vi "GetLinkerDependencyFromFiles.vi"(9 "Overwrite LabVIEW Folder(If empty use this version of LabVIEW)":path, 10 "MaxDepth(<=0 No limit)":i32=-1, 11 "All Files in Dir":path[](array[path])) -> (3 "FileDependency":map{path, T1}(c390))   [LabVIEW 2020, in "DependencyViewer.lvlib"]
uses:
  DependencyViewer.lvlib
  FileDependencyType.ctl
  <vilib>/Utility/lvfile.llb/FT_FileTypes.ctl
  fa84a50a-7a91-41f1-93a7-6c8b41b91fd3.vi
  <vilib>/Utility/lvfile.llb/NI_FileType.lvlib
panel:
  out "Dependecy":T1
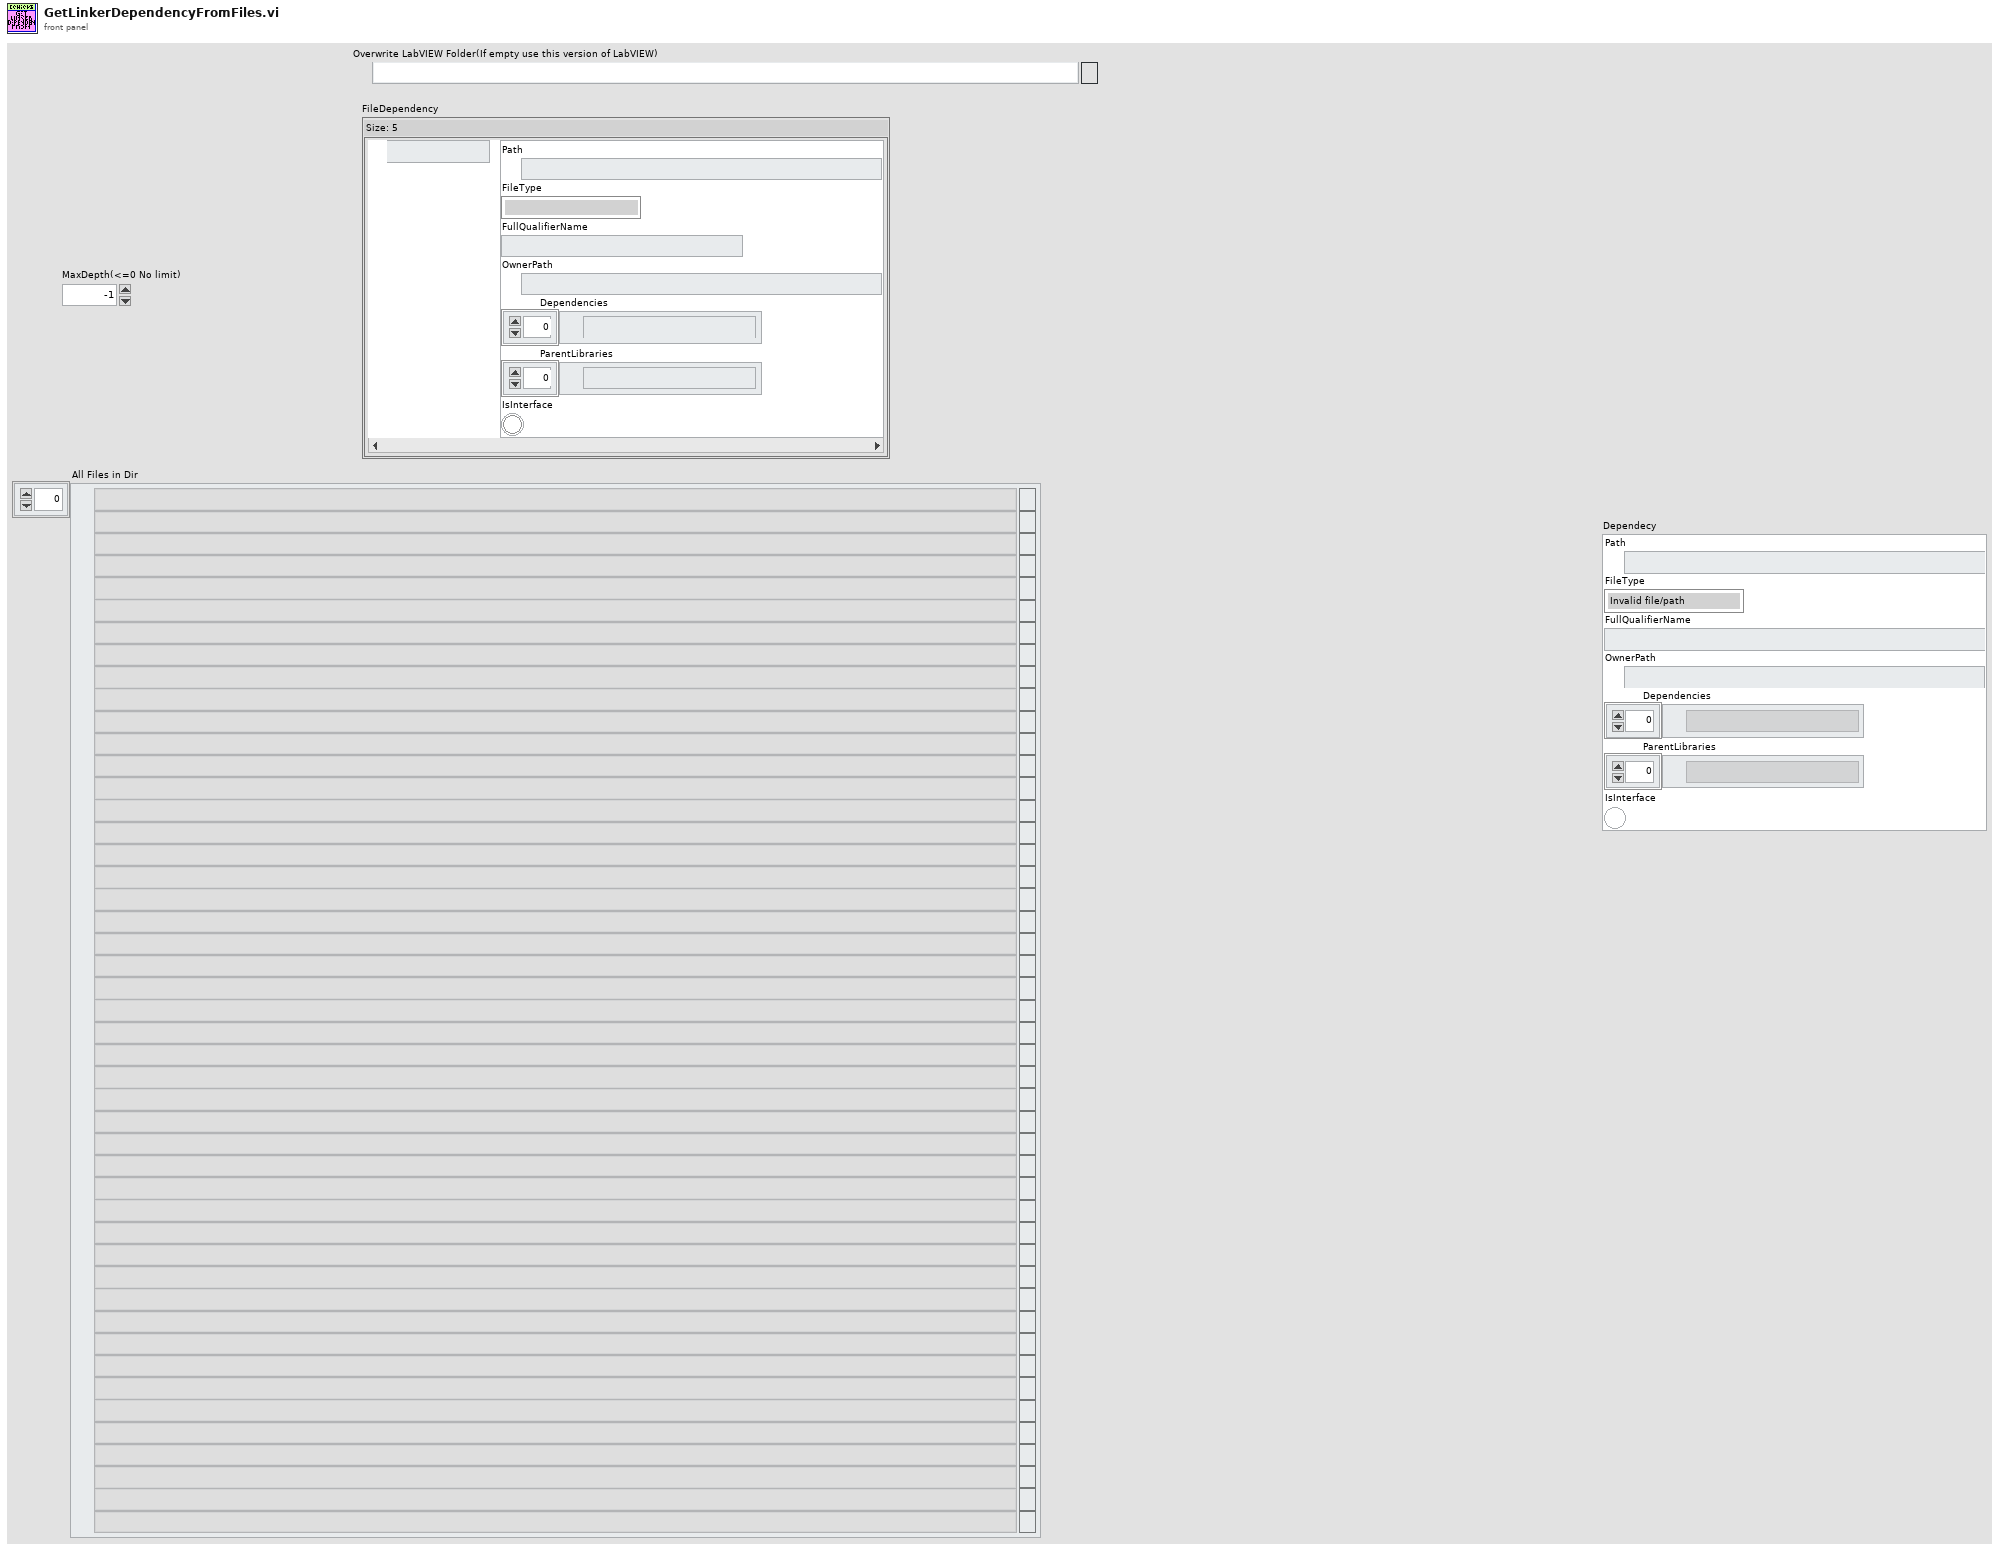
[diagram p1: front panel]
types:
  T1 = typedef "DependencyViewer.lvlib/FileDependencyType.ctl" = cluster{"Path":path, "FileType":T2, "FullQualifierName":string, "OwnerPath":path, "Dependencies":path[], "ParentLibraries":path[], "IsInterface":bool}
  T2 = typedef "NI_FileType.lvlib/FT_FileTypes.ctl" = enum32{"Invalid file/path", "Unknown type", "Instrument", "Control", "Polymorphic VI", "Project", "Library", "LVClass", "XControl", "XNode", "CIN", "Run-time menu", "Palette menu", "LLB", "Shortcut", "Directory", "Class Private Data Control", "Statechart", "MathScript .m file", "Ladder Diagram", "LVLibp"}
  T3 = typedef "NI_FileType.lvlib/LVFileType.ctl" = enum32{"Invalid file", "Unknown type", "Instrument", "Control", "Polymorphic VI", "Project", "Library", "LVClass", "XControl", "XNode", "Shared library", ".NET assembly", "ActiveX interface", "CIN", "Run-time menu", "Palette menu", "Help file", "LLB", "XNode Edit Dependency", "Class Private Data Control", "Statechart", "MathScript .m file", "Ladder Diagram", "LVLibp", "XNode Build Dependency"}
  T4 = cluster{"path":path, "delimited name":string, "type":T3, "iState":u32, "iStyle":u16, "wStyle":u16, "buttons":u16, "viflags":u32, "viflags2":u32, "links":u32[]}[]
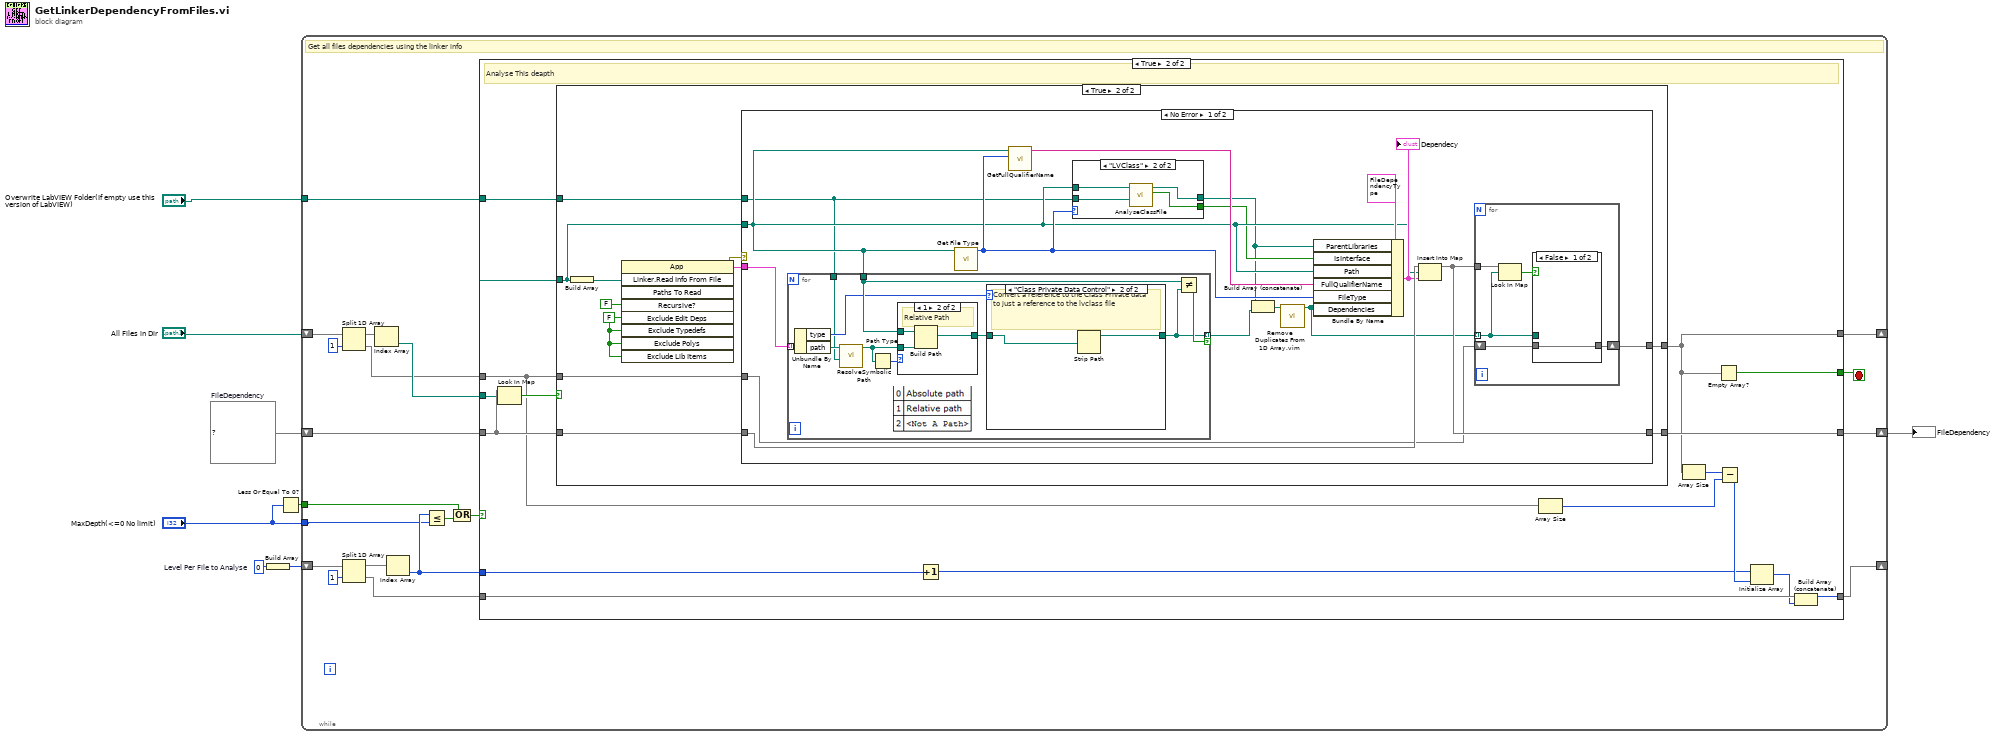
[diagram p0: block diagram]
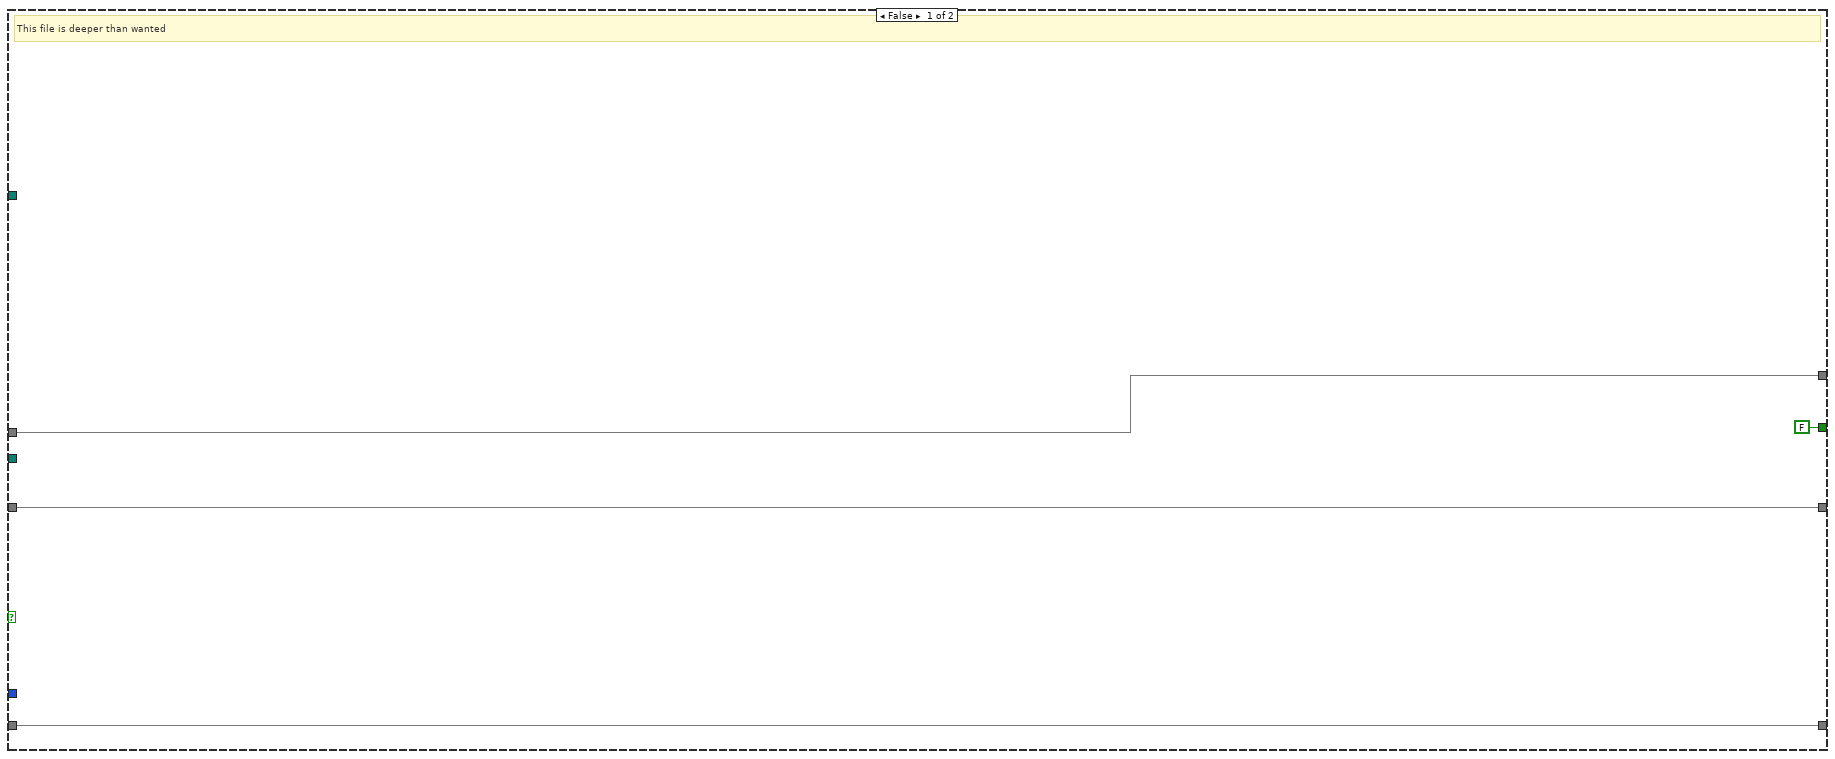
[diagram p2: hidden frame]
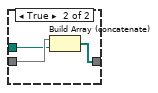
[diagram p5: hidden frame]
diagram:
  w4 = 0  # Level Per File to Analyse
  w7 = map{path, T1} {}  # FileDependency
  n1 = Build Array(w4) -> (w3:i32[])
  n2 = Less Or Equal To 0?(x="MaxDepth(<=0 No limit)") -> (x <= 0?=w1:bool)
  n3 = while {
    shift-right: [w25] -> w8
    shift-left: w7 -> [w24]
    shift-right: [w16] -> _
    shift-left: "All Files in Dir" -> [w28]
    tunnel: "Overwrite LabVIEW Folder(If empty use this version of LabVIEW)" -> [w22]
    tunnel: "MaxDepth(<=0 No limit)" -> [w12]
    shift-right: [w14] -> _
    shift-left: w3 -> [w20]
    tunnel: w1 -> [w9]
    stop <- w19 stop-if-true
    # "Get all files dependencies using the linker info"
    n4 = Split 1D Array(array=w28, index=1) -> (first subarray=w26:path[], second subarray=w17:path[])
    n5 = Split 1D Array(array=w20, index=1) -> (first subarray=w18:i32[], second subarray=w15:i32[])
    n6 = Index Array(array=w26) -> (element=w23:path)  [unwired: 1 in]
    n7 = Index Array(array=w18) -> (element=w13:i32)  [unwired: 1 in]
    n8 = Less Or Equal?(x=w13, y=w12) -> (x <= y?=w11:bool)
    n9 = Compound Arithmetic op=OR(w9, w11) -> (w10:bool)
    n10 = case shown="True" w10 {
      tunnel: [w30 w48] -> w25
      tunnel: w24 -> [w30 w47]
      tunnel: w23 -> [_ w45]
      tunnel: w22 -> [_ w44]
      tunnel: [FALSE ("empty?") w43] -> w19
      tunnel: w17 -> [w32 w42]
      tunnel: [w32 w41] -> w16
      tunnel: w15 -> [w31 w36]
      tunnel: [w31 w34] -> w14
      tunnel: w13 -> [_ w33]
      frame False {
        # "This file is deeper than wanted"
      }
      frame True {
        # "Analyse This deapth"
        n11 = Look In Map(map=w47, key=w45) -> (key not found?=w46:bool)  [unwired: 1 in, 1 out]
        n12 = case shown="True" w46 {
          tunnel: w42 -> [w49 w61]
          tunnel: [w50 w60] -> w48
          tunnel: [w49 w59] -> w41
          tunnel: w47 -> [w50 w54]
          tunnel: w45 -> [_ w53]
          tunnel: w44 -> [_ w51]
          frame False {
          }
          frame True {
            w52 = FALSE ("Exclude Edit Time Dependencies")
            n13 = Build Array(w53) -> (w58:path[])
            n14 = invoke class="App" method="Linker.Read Info From File"("Paths To Read"=w58, "Recursive?"=FALSE, "Exclude Edit Deps"=w52, "Exclude Typedefs"=w52, "Exclude Polys"=w52, "Exclude Lib Items"=w52) -> (error out=w55:errorcluster, "Linker.Read Info From File"=w56:T4)  [unwired: 3 in, 7 out]
            n15 = case shown="No Error" w55 {
              tunnel: w56 -> [w76 _]
              tunnel: w54 -> [w77 w108]
              tunnel: w61 -> [w73 w109]
              tunnel: [w72 w109] -> w59
              tunnel: w53 -> [w67 _]
              tunnel: [w74 w108] -> w60
              tunnel: w51 -> [w62 _]
              frame No Error {
                n16 = for {
                  tunnel: w76 -> [w100] mode=indexing
                  tunnel: [w92] -> w68 mode=indexing if=w97
                  tunnel: w67 -> [w96]
                  tunnel: w62 -> [w91]
                  n17 = Unbundle By Name(w100) -> ("type"=w94:T3, "path"=w98:path)
                  n18 = call "ResolveSymbolicPath.vi"("Overwrite LabVIEW Folder(If empty use this version of LabVIEW)"=w91, "path"=w98) -> ("File Path"=w95:path)  [unwired: 9 in]
                  n19 = Path Type(1:w95) -> (0:w99:i16)
                  n20 = case shown="1" w99 {
                    tunnel: w95 -> [w104 w107]
                    tunnel: [w104 w105] -> w93
                    tunnel: w96 -> [_ w106]
                    frame 0, Default {
                      # "Absolute Path"
                    }
                    frame 1 {
                      # "Relative Path"
                      n21 = Build Path(base path=w106, name or relative path=w107) -> (appended path=w105:path)
                    }
                  }
                  n22 = case shown="\"Class Private Data Control\"" w94 {
                    tunnel: w93 -> [w101 w103]
                    tunnel: [w101 w102] -> w92
                    frame Default {
                    }
                    frame "Class Private Data Control" {
                      # "Convert a reference to the Class Private data to just a reference to the lvclass file"
                      n23 = Strip Path(path=w103) -> (stripped path=w102:path)  [unwired: 1 out]
                    }
                  }
                  n24 = Not Equal?(x=w96, y=w92) -> (x != y?=w97:bool)
                }
                n25 = call <vilib>:"Get File Type.vi"("path"=w67) -> ("file type"=w70:T2)  [unwired: 8 in, 2 out]
                n26 = call "GetFullQualifierName.vi"("file type"=w70, "File Path"=w67) -> ("FullQualifierName"=w71:string)  [unwired: 9 in]
                n27 = case shown="\"LVClass\"" w70 {
                  tunnel: w67 -> [_ w81]
                  tunnel: [_ w80] -> w65
                  tunnel: [_ w79] -> w66
                  tunnel: w62 -> [_ w78]
                  frame "Invalid file/path", Default {
                  }
                  frame "LVClass" {
                    n28 = call "AnalyseClassFile.vi"("Overwrite LabVIEW Folder(If empty use this version of LabVIEW)"=w78, "File Path"=w81) -> ("IsInterface"=w79:bool, "ParentLibraries"=w80:path[])  [unwired: 8 in]
                  }
                }
                n29 = Build Array (concatenate)(w65, w68) -> (w64:path[])
                n30 = call "Remove Duplicates From 1D Array.vim"("array"=w64) -> ("array with duplicates removed"=w63:path[])  [unwired: 10 in]
                n31 = Bundle By Name(cluster=T1 {"Path"=path "", "FileType"=enum."Instrument", "FullQualifierName"="Decorator1_Main.vi", "OwnerPath"=path "", "Dependencies"=[], "ParentLibraries"=[], "IsInterface"=FALSE} ("value"), "ParentLibraries"=w65, "IsInterface"=w66, "Path"=w67, "FullQualifierName"=w71, "FileType"=w70, "Dependencies"=w63) -> (w75:T1)
                "Dependecy" <- w75
                n32 = Insert Into Map(map in=w77, key=w67, value=w75) -> (map out=w74:map{path, T1})  [unwired: 2 out]
                n33 = for {
                  tunnel: w74 -> [w86]
                  tunnel: w63 -> [w82] mode=indexing
                  shift-right: [w83] -> w72
                  shift-left: w73 -> [w84]
                  n34 = Look In Map(map=w86, key=w82) -> (key not found?=w85:bool)  [unwired: 1 in, 1 out]
                  n35 = case shown="False" w85 {
                    tunnel: w84 -> [w87 w90]
                    tunnel: [w87 w89] -> w83
                    tunnel: w82 -> [_ w88]
                    frame False {
                    }
                    frame True {
                      n36 = Build Array (concatenate)(w90, w88) -> (w89:path[])
                    }
                  }
                }
              }
              frame Error {
              }
            }
          }
        }
        n37 = Increment(x=w33) -> (x+1=w37:i32)
        n38 = Array Size(array=w42) -> (size(s)=w39:i32)
        n39 = Array Size(array=w41) -> (size(s)=w40:i32)
        n40 = Empty Array?(array=w41) -> (empty?=w43:bool)
        n41 = Subtract(x=w40, y=w39) -> (x-y=w38:i32)
        n42 = Initialize Array(w37, w38) -> (w35:i32[])
        n43 = Build Array (concatenate)(w36, w35) -> (w34:i32[])
      }
    }
  }
  "FileDependency" <- w8
